vi "getPosServos.vi"(0 "channel":u8 max=15 step=1) -> (1 "position":u16, 2 "return count":u32)   [LabVIEW 2011]
uses:
  GlobalSerial.vi
panel:
  out "channel":u8
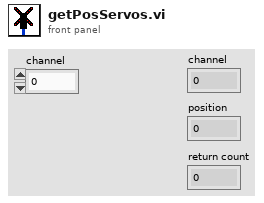
[diagram p1: front panel]
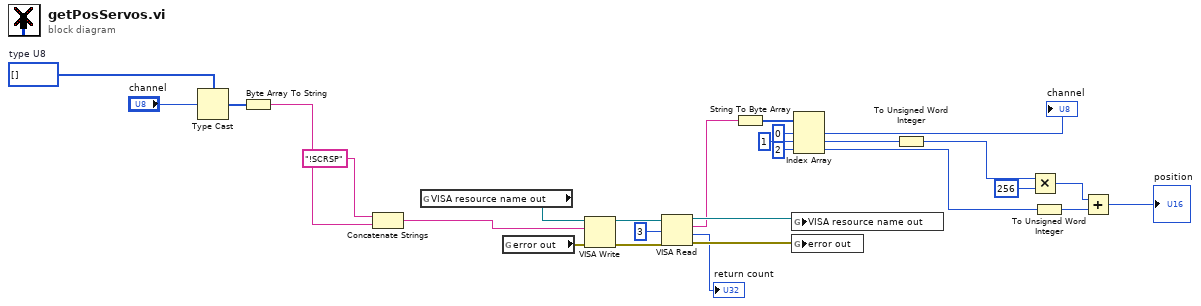
[diagram p0: block diagram]
diagram:
  w23 = u8[] []  # type U8
  n1 = Type Cast(type=w23, x="channel") -> (*(type *) &x=w25:u8[])
  n2 = Byte Array To String(unsigned byte array=w25) -> (string=w26:string)
  n3 = Concatenate Strings("!SCRSP" ("string"), w26) -> (w22:string)
  n4 = global read "GlobalSerial.vi" "VISA resource name out"() -> (w20:refnum<visa-resource-name>)
  n5 = global read "GlobalSerial.vi" "error out"() -> (w21:errorcluster)
  n6 = VISA Write(VISA resource name=w20, write buffer=w22, error in (no error)=w21) -> (VISA resource name out=w19:refnum<visa-resource-name>, error out=w18:errorcluster)  [unwired: 1 out]
  n7 = VISA Read(VISA resource name=w19, byte count=u32 3, error in (no error)=w18) -> (VISA resource name out=w16:refnum<visa-resource-name>, read buffer=w13:string, return count=→"return count":u32, error out=w17:errorcluster)
  n8 = String To Byte Array(string=w13) -> (unsigned byte array=w12:u8[])
  n9 = global write "GlobalSerial.vi" "VISA resource name out"(w16) -> ()
  n10 = global write "GlobalSerial.vi" "error out"(w17) -> ()
  n11 = Index Array(array=w12, index #1=0 ("index"), index #2=1 ("index"), index #3=2 ("index")) -> (element #1=→"channel":u8, element #2=w2:u8, element #3=w3:u8)
  n12 = To Unsigned Word Integer(number=w2) -> (unsigned 16bit integer=w7:u16)
  n13 = Multiply(x=w7, y=u16 256) -> (x*y=w5:u16)
  n14 = To Unsigned Word Integer(number=w3) -> (unsigned 16bit integer=w4:u16)
  n15 = Add(x=w5, y=w4) -> (x+y=→"position":u16)
